vi "FTW-Endpoint-TCP-Reply-Send-Worker-Start.vi"(0 "FTW-Endpoint-TCP In":refnum<class "FTW-Endpoint-TCP.lvclass">, 11 "error in":errorcluster) -> (4 "FTW-Endpoint-TCP Out":refnum<class "FTW-Endpoint-TCP.lvclass">, 15 "error out":errorcluster)   [LabVIEW 2015, in "FTW-Endpoint-TCP.lvclass"]
uses:
  FTW-Endpoint-TCP.lvclass
  FTW-Endpoint-TCP-Reply-Send-Worker.vi
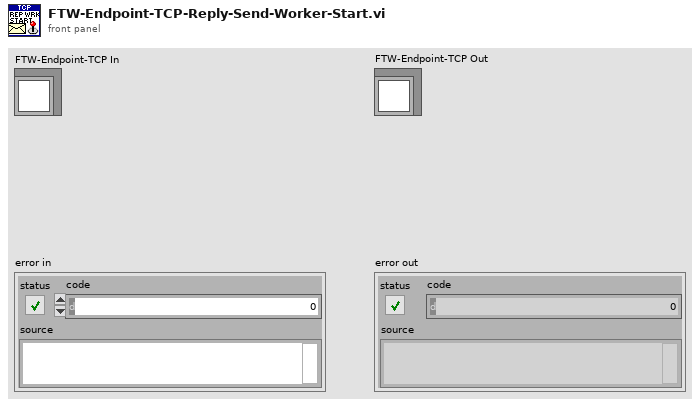
[diagram p1: front panel]
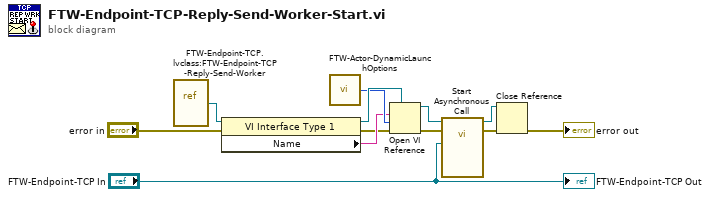
[diagram p0: block diagram]
diagram:
  n1 = vi-ref "FTW-Endpoint-TCP.lvclass:FTW-Endpoint-TCP-Reply-Send-Worker.vi"() -> (w1:refnum<vi>)
  n2 = property class="VI Interface Type 1"(reference=w1, error in="error in") -> (reference out=w5:refnum<vi>, error out=w2:errorcluster, "Name"=w3:string)
  n3 = call "FTW-Actor-DynamicLaunchOptions.vi"() -> ("Open VI Ref Options"=w4:i32)
  n4 = Open VI Reference(type specifier VI Refnum (for type only)=w5, vi path=w3, options=w4, error in (no error)=w2) -> (vi reference=w7:refnum<vi>, error out=w9:errorcluster)  [unwired: 2 in]
  n5 = call-by-ref "Start Asynchronous Call"(reference=w7, error in=w9, "TCP Endpoint"="FTW-Endpoint-TCP In") -> (reference out=w8:refnum<vi>, error out=w6:errorcluster)  [unwired: 15 in]
  n6 = Close Reference(reference=w8, error in (no error)=w6) -> (error out=→"error out":errorcluster)
  "FTW-Endpoint-TCP Out" <- "FTW-Endpoint-TCP In"
